vi "ChannelCore CreateFIFOInstance.vi"(6 "contextId":T1, 8 "error in":errorcluster, 9 "timeout (ms)":i32=-1, 10 "Request Data":T4, 11 "gRPC ID":T1) -> (0 "error out":errorcluster, 2 "Response Data":T2, 3 "gRPC ID out":T1)   [LabVIEW 2021, in "CIFCoreChannel_client.lvlib"]
uses:
  CIFCoreChannel_client.lvlib
  <vilib>/gRPC/LabVIEW gRPC Library/Shared/grpcId.ctl
  RPC Messages/cif_channelcore_FIFOInstance.ctl
  RPC Messages/cif_channelcore_FIFOReference.ctl
  RPC Messages/cif_common_Status.ctl
  RPC Messages/cif_channelcore_FIFOReference_Flat.ctl
  RPC Messages/cif_common_Status_Flat.ctl
  14035477-4c25-4107-8ed5-d0c4ef420ce5.vi
  <vilib>/gRPC/LabVIEW gRPC Library/Shared/TranslateGrpcError.vi
  <vilib>/gRPC/LabVIEW gRPC Library/Shared/Wait On Occurrence.vi
  RPC Messages/FlatToRichcif_common_Status.vi
  <vilib>/gRPC/LabVIEW gRPC Library/Shared/Is Feature Enabled.vi
  <vilib>/gRPC/LabVIEW gRPC Library/Server API/Server/Get Server DLL Path.vi
  <vilib>/Utility/error.llb/Error Cluster From Error Code.vi
  <vilib>/gRPC/LabVIEW gRPC Library/grpc-lvsupport-release.lvlib
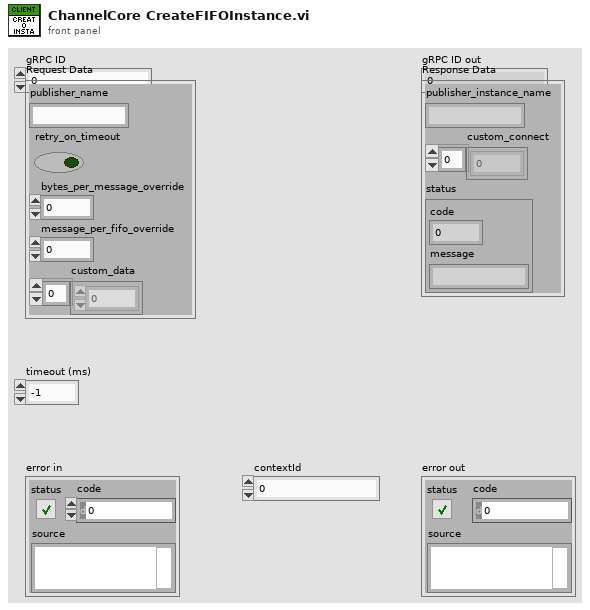
[diagram p1: front panel]
types:
  T1 = typedef "grpc-lvsupport-release.lvlib/grpcId.ctl" = u64
  T2 = typedef "CIFCoreChannel_client.lvlib/cif_channelcore_FIFOReference.ctl" = cluster{"publisher_instance_name":string, "custom_connect":u8[], "status":T3}
  T3 = typedef "CIFCoreChannel_client.lvlib/cif_common_Status.ctl" = cluster{"code":i32, "message":string}
  T4 = typedef "CIFCoreChannel_client.lvlib/cif_channelcore_FIFOInstance.ctl" = cluster{"publisher_name":string, "retry_on_timeout":bool, "bytes_per_message_override":u32, "message_per_fifo_override":u32, "custom_data":u8[]}
  T5 = typedef "CIFCoreChannel_client.lvlib/cif_channelcore_FIFOReference_Flat.ctl" = cluster{"publisher_instance_name":string, "custom_connect":u8[], "status":T6}
  T6 = typedef "CIFCoreChannel_client.lvlib/cif_common_Status_Flat.ctl" = cluster{"code":i32, "message":string}
  T7 = typedef "CIFCoreChannel_client.lvlib/cif_channelcore_FIFOInstance_Flat.ctl" = cluster{"publisher_name":string, "retry_on_timeout":bool, "bytes_per_message_override":u32, "message_per_fifo_override":u32, "custom_data":u8[]}
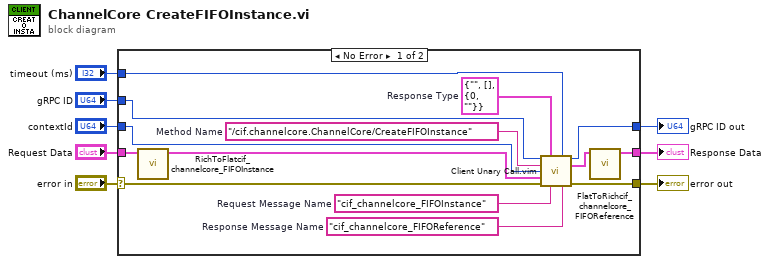
[diagram p0: block diagram]
diagram:
  n1 = case shown="No Error" "error in" {
    selector: "error in" -> [w18 w23]
    tunnel: [w17 w23] -> w7
    tunnel: "gRPC ID" -> [w16 w24]
    tunnel: [w15 w24] -> w5
    tunnel: "Request Data" -> [w12 _]
    tunnel: [w9 _] -> w3
    tunnel: "timeout (ms)" -> [w14 _]
    tunnel: "contextId" -> [w13 _]
    frame No Error {
      w19 = "cif_channelcore_FIFOReference"  # Response Message Name
      w20 = "cif_channelcore_FIFOInstance"  # Request Message Name
      w21 = T5 {"publisher_instance_name"="", "custom_connect"=[], "status"={"code"=0, "message"=""}}  # Response Type
      w22 = "/cif.channelcore.ChannelCore/CreateFIFOInstance"  # Method Name
      n2 = call "RichToFlatcif_channelcore_FIFOInstance.vi"("InputCluster"=w12) -> ("OutputCluster"=w11:T7)  [unwired: 10 in]
      n3 = call "Client Unary Call.vim"("ClientID in"=w16, "Response Type"=w21, "timeout (ms)"=w14, "Method Name"=w22, "contextId"=w13, "Request Data"=w11, "error in"=w18, "Request Message Name"=w20, "Response Message Name"=w19) -> ("ClientID out"=w15:u64, "Response Data"=w10:T5, "error out"=w17:errorcluster)  [unwired: 4 in]
      n4 = call "FlatToRichcif_channelcore_FIFOReference.vi"("InputCluster"=w10) -> ("OutputCluster"=w9:T2)  [unwired: 10 in]
    }
    frame Error {
    }
  }
  "error out" <- w7
  "gRPC ID out" <- w5
  "Response Data" <- w3
